vi "getadminpassword.vi"() -> (0 "Password":string)   [LabVIEW 2024]
uses:
  <vilib>/drjdpowell/SQLite Library/SQL Connection/Connection.lvclass
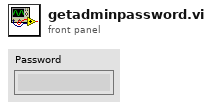
[diagram p1: front panel]
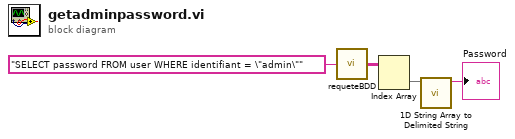
[diagram p0: block diagram]
diagram:
  n1 = call "requeteBDD.vi"("Requête Sql"="SELECT password FROM user WHERE identifiant = \"admin\"" ("SQL")) -> ("Table Control"=w1:string[][])
  n2 = Index Array(array=w1) -> (element=w3:string[])  [unwired: 2 in]
  n3 = call <vilib>:"1D String Array to Delimited String.vi"("string array"=w3) -> ("delimited string"=→"Password":string)  [unwired: 10 in]
